vi "Print.vi"(8 "error in":errorcluster, 11 "OD Entry in":refnum<class "OD Entry.lvclass">) -> (0 "error out":errorcluster, 2 "Entry with Sub-Entries":map{string, string}[](array[numeric]), 3 "OD Entry out":refnum<class "OD Entry.lvclass">)   [LabVIEW 2024, in "Electronic Datasheet.lvlib" / "OD Entry.lvclass"]
uses:
  OD Entry.lvclass
  OD Sub-Entry/OD Sub-Entry.lvclass
  D:/git/EDS-File-Viewer/source/Core/OD Entry/OD Entry.lvclass
  Object Type/Object Type Base.lvclass
  OD Entry.lvclass/OD Entry.ctl
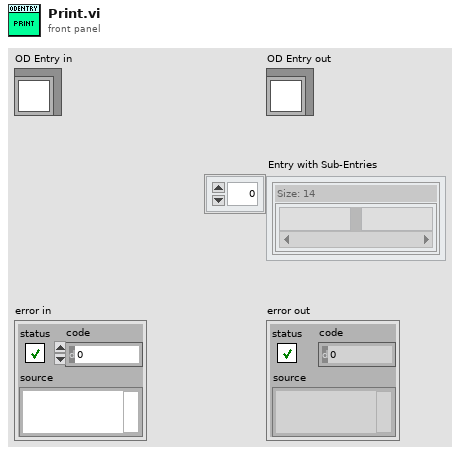
[diagram p1: front panel]
types:
  T1 = typedef "Electronic Datasheet.lvlib/OD Entry.lvclass/ObjectAttributes.ctl" = cluster{"Index":u16, "ObjectType":refnum<class "Object Type Base.lvclass">, "Denotation":string, "Count":u8, "ObjExtend":u8, "Label":string, "Description":string, "PDO Mapping Type":T2, "Sub-Entries":map{u8, refnum<class "OD Sub-Entry.lvclass">}}
  T2 = typedef "Electronic Datasheet.lvlib/PDO Mapping Type.ctl" = enum16{"no", "optional", "RPDO", "TPDO", "UNKNOWN"}
  T3 = typedef "Electronic Datasheet.lvlib/Access SDO.ctl" = enum16{"read only", "write only", "read/write", "read/write on process input", "read/write on process output", "constant value", "no", "UNKNOWN"}
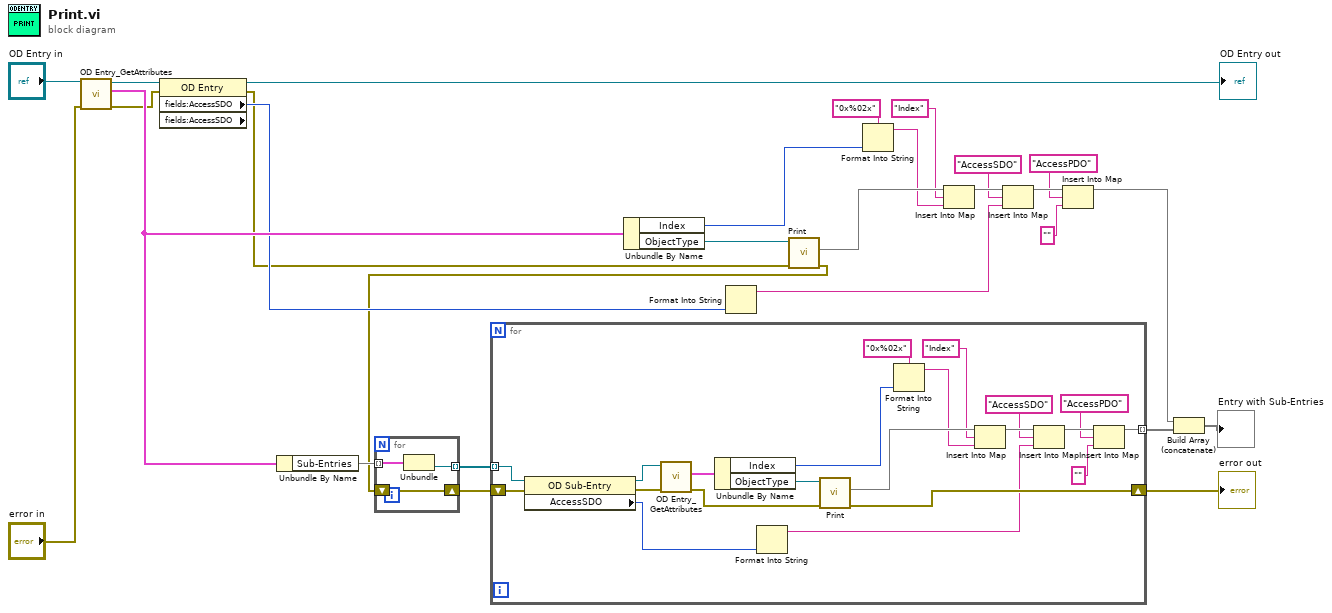
[diagram p0: block diagram]
diagram:
  n1 = call "OD Entry_GetAttributes.vi"("Error In"="error in", "reference in"="OD Entry in") -> ("Error Out"=w7:errorcluster, "Data"=w19:T1, "reference out"=w27:refnum<class "OD Entry.lvclass">)  [unwired: 6 in, 1 out]
  n2 = property class="OD Entry" props=["fields:AccessSDO", "fields:AccessSDO"](reference=w27, error in=w7) -> (reference out=→"OD Entry out":refnum<class "OD Entry.lvclass">, error out=w3:errorcluster, "fields:AccessSDO"=w6:T3)  [unwired: 1 out]
  n3 = Unbundle By Name(w19) -> ("Sub-Entries"=w25:map{u8, refnum<class "OD Sub-Entry.lvclass">})
  n4 = Unbundle By Name(w19) -> ("Index"=w5:u16, "ObjectType"=w4:refnum<class "Object Type Base.lvclass">)
  n5 = Format Into String(w6) -> (resulting string=w11:string)  [unwired: 3 in, 1 out]
  n6 = call-dynamic "Print.vi"("error in"=w3, "Object Type Base in"=w4) -> ("error out"=w2:errorcluster, "Fields"=w17:map{string, string})  [unwired: 7 in, 1 out]
  n7 = for {
    tunnel: w25 -> [w31] mode=indexing
    tunnel: [w29] -> w24 mode=indexing
    shift-right: [w30] -> w23
    shift-left: w2 -> [w30]
    n8 = Unbundle(w31) -> ("OD Sub-Entry"=w29:refnum<class "OD Sub-Entry.lvclass">)  [unwired: 1 out]
  }
  n9 = for {
    tunnel: w24 -> [w45] mode=indexing
    shift-right: [w47] -> w21
    shift-left: w23 -> [w46]
    tunnel: [w34] -> w22 mode=indexing
    n10 = property class="OD Sub-Entry"(reference=w45, error in=w46) -> (reference out=w43:refnum<class "OD Sub-Entry.lvclass">, error out=w44:errorcluster, "AccessSDO"=w36:T3)
    n11 = call "OD Entry_GetAttributes.vi"("Error In"=w44, "reference in"=w43) -> ("Error Out"=w39:errorcluster, "Data"=w42:T1)  [unwired: 6 in, 2 out]
    n12 = Unbundle By Name(w42) -> ("Index"=w40:u16, "ObjectType"=w41:refnum<class "Object Type Base.lvclass">)
    n13 = Format Into String(w36) -> (resulting string=w35:string)  [unwired: 3 in, 1 out]
    n14 = call-dynamic "Print.vi"("error in"=w39, "Object Type Base in"=w41) -> ("error out"=w47:errorcluster, "Fields"=w51:map{string, string})  [unwired: 7 in, 1 out]
    n15 = Format Into String(format string="0x%02x", w40) -> (resulting string=w50:string)  [unwired: 2 in, 1 out]
    n16 = Insert Into Map(map in=w51, key="Index", value=w50) -> (map out=w48:map{string, string})  [unwired: 2 out]
    n17 = Insert Into Map(map in=w48, key="AccessSDO", value=w35) -> (map out=w38:map{string, string})  [unwired: 2 out]
    n18 = Insert Into Map(map in=w38, key="AccessPDO", value="") -> (map out=w34:map{string, string})  [unwired: 2 out]
  }
  "error out" <- w21
  n19 = Format Into String(format string="0x%02x", w5) -> (resulting string=w16:string)  [unwired: 2 in, 1 out]
  n20 = Insert Into Map(map in=w17, key="Index", value=w16) -> (map out=w14:map{string, string})  [unwired: 2 out]
  n21 = Insert Into Map(map in=w14, key="AccessSDO", value=w11) -> (map out=w13:map{string, string})  [unwired: 2 out]
  n22 = Insert Into Map(map in=w13, key="AccessPDO", value="") -> (map out=w1:map{string, string})  [unwired: 2 out]
  n23 = Build Array (concatenate)(w1, w22) -> (→"Entry with Sub-Entries":map{string, string}[])
